vi "test Counter Data Plugin Run.vi"(8 "error in (no error)":errorcluster, 11 "TestCase in":refnum<class "Data Engine Unit Tests.lvclass">) -> (0 "error out":errorcluster, 3 "TestCase out":refnum<class "Data Engine Unit Tests.lvclass">)   [LabVIEW 2017, in "Data Engine Unit Tests.lvclass"]
uses:
  Data Engine Unit Tests.lvclass
  Source/Counter Data Plugin/Counter Data Plugin.lvclass
  D:/xtra/vi/Data Engine/Data Plugin/Data Plugin.lvclass
  <vilib>/addons/_JKI Toolkits/VI Tester/TestCase.llb/TestCase.lvclass
  C:/Program Files/National Instruments/LabVIEW 2017/vi.lib/addons/_JKI Toolkits/VI Tester/TestCase.llb/TestCase.lvclass
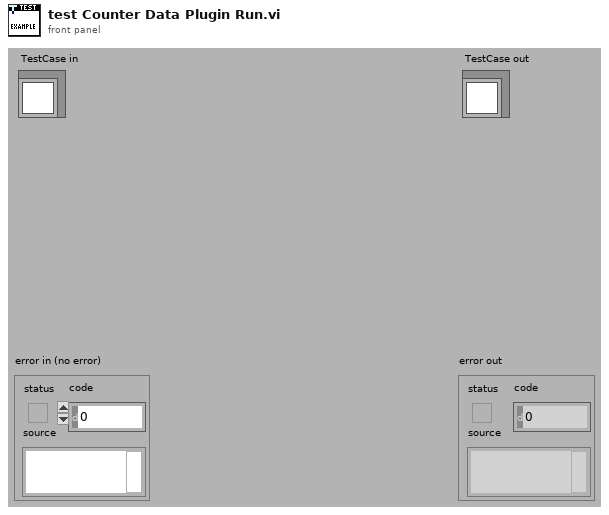
[diagram p1: front panel]
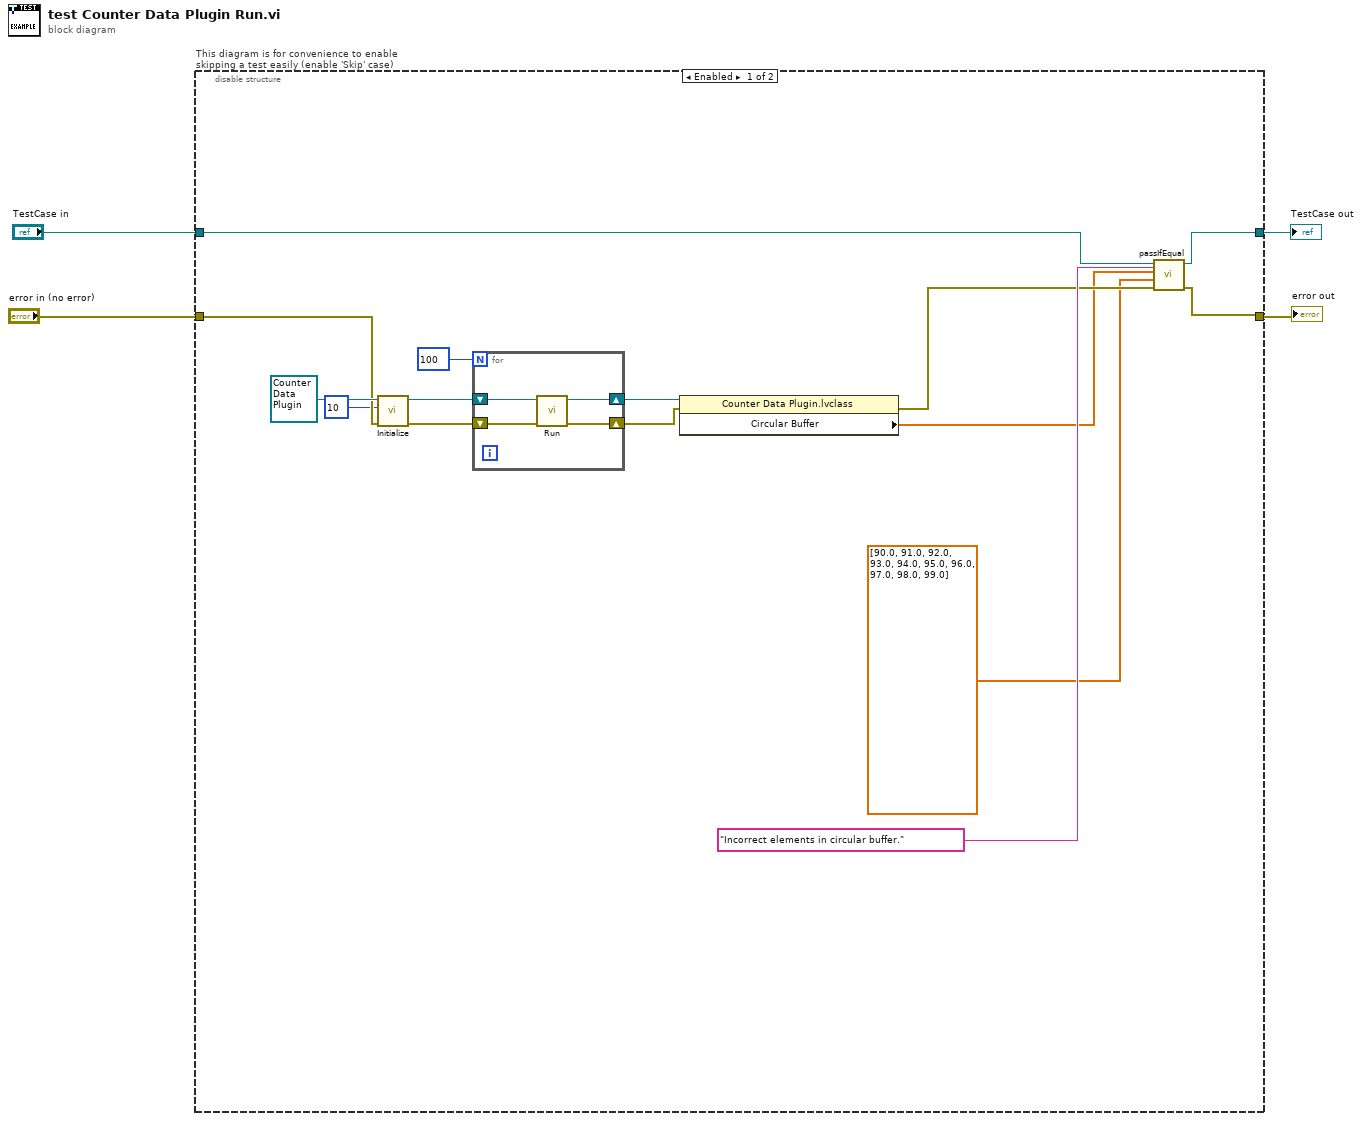
[diagram p0: block diagram]
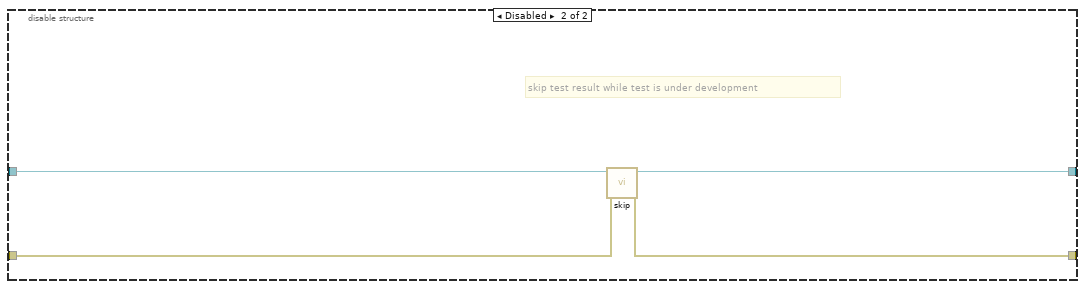
[diagram p2: hidden frame]
diagram:
  n1 = disable-structure "This diagram is for convenience to enable skipping a test easily (enable 'Skip' case)" shown="Enabled" {
    disable-tunnel: "TestCase in" -> [w5 w27]
    disable-tunnel: [w11 w25] -> w1
    disable-tunnel: [w10 w26] -> w3
    disable-tunnel: "error in (no error)" -> [w18 w24]
    frame Enabled {
      n2 = call-dynamic "Initialize.vi"("error in (no error)"=w18, "Circular Buffer Size"=10, "Data Plugin in"=refnum<class "Counter Data Plugin.lvclass"> refnum ("Data Engine.lvlib:Counter Data Plugin.lvclass")) -> ("error out"=w17:errorcluster, "Data Plugin out"=w16:refnum<class "Counter Data Plugin.lvclass">)  [unwired: 7 in]
      n3 = for {
        N: 100 -> [_]
        shift-right: [w22] -> w13
        shift-left: w17 -> [w23]
        shift-right: [w20] -> w14
        shift-left: w16 -> [w21]
        n4 = call-dynamic "Run.vi"("error in (no error)"=w23, "Data Plugin in"=w21) -> ("error out"=w22:errorcluster, "Data Plugin out"=w20:refnum<class "Counter Data Plugin.lvclass">)  [unwired: 8 in]
      }
      n5 = property class="Counter Data Plugin.lvclass"(reference=w14, error in=w13) -> (error out=w8:errorcluster, "Circular Buffer"=w7:dbl[])  [unwired: 1 out]
      n6 = call-dynamic "passIfEqual.vi"("custom report message (\"\")"="Incorrect elements in circular buffer." ("message (\"\")"), "error in (no error)"=w8, "y"=dbl[] [90.0, 91.0, 92.0, 93.0, 94.0, 95.0, 96.0, 97.0, 98.0, 99.0], "x"=w7, "TestCase in"=w5) -> ("error out"=w10:errorcluster, "TestCase out"=w11:refnum<class "Data Engine Unit Tests.lvclass">)  [unwired: 5 in]
    }
    frame Disabled {
      # "skip test result while test is under development"
      n7 = call <vilib>:"skip.vi"("error in (no error)"=w24, "TestCase in"=w27) -> ("error out"=w26:errorcluster, "TestCase out"=w25:refnum<class "Data Engine Unit Tests.lvclass">)  [unwired: 8 in]
    }
  }
  "error out" <- w3
  "TestCase out" <- w1
